vi "ClearListBox.vi"(8 "error in (no error)":errorcluster, 11 "GUI_Handler_Seq in":refnum<class "GUI_Handler_Seq.lvclass">) -> (0 "error out":errorcluster, 3 "GUI_Handler_Seq out":refnum<class "GUI_Handler_Seq.lvclass">)   [LabVIEW 2019, in "GUI_Handler_Seq.lvclass"]
uses:
  GUI_Handler_Seq.lvclass
  <vilib>/Utility/miscctls.llb/LVRowAndColumnTypeDef.ctl
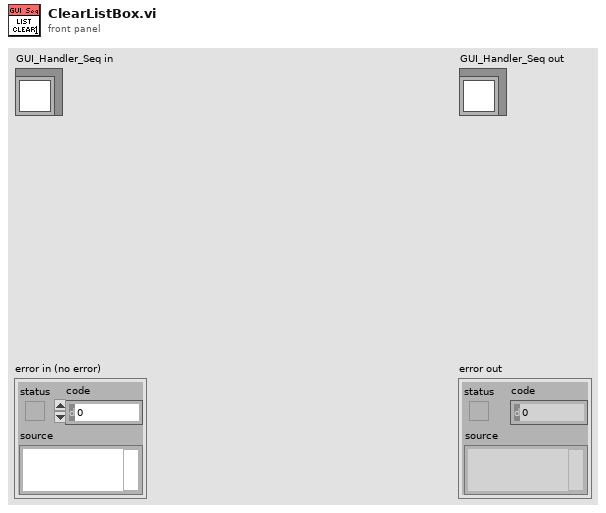
[diagram p1: front panel]
types:
  T1 = typedef "LVRowAndColumnTypeDef.ctl" = cluster{"Row":i32, "Column":i32}
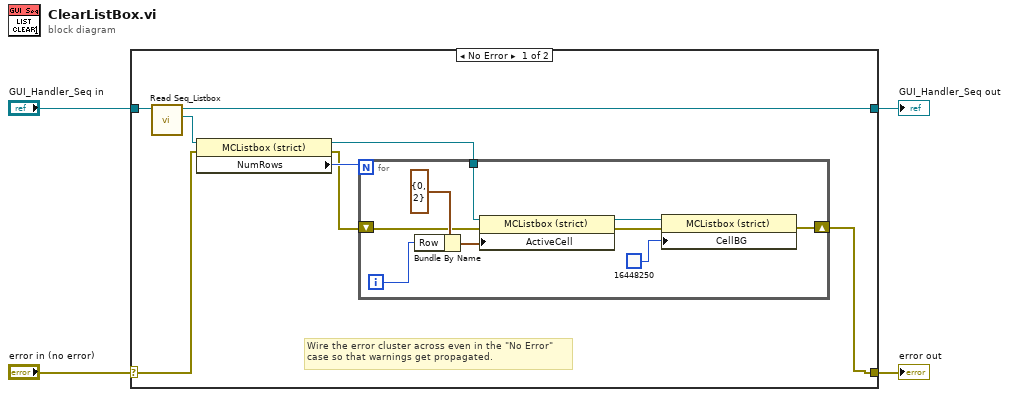
[diagram p0: block diagram]
diagram:
  n1 = case shown="No Error" "error in (no error)" {
    selector: "error in (no error)" -> [w6 w22]
    tunnel: [w5 w22] -> w1
    tunnel: [w12 w23] -> w2
    tunnel: "GUI_Handler_Seq in" -> [w11 w23]
    frame No Error {
      # "Wire the error cluster across even in the \"No Error\"\ncase so that warnings get propagated."
      n2 = call-dynamic "Read Seq_Listbox.vi"("GUI_Handler_Seq in"=w11) -> ("Seq_Listbox"=w10:refnum<vi>, "GUI_Handler_Seq out"=w12:refnum<class "GUI_Handler_Seq.lvclass">)  [unwired: 8 in, 1 out]
      n3 = property class="MCListbox (strict)"(reference=w10, error in=w6) -> (reference out=w8:refnum<vi>, error out=w7:errorcluster, "NumRows"=w9:u32)
      n4 = for {
        N: w9 -> [_]
        tunnel: w8 -> [w18]
        shift-right: [w14] -> w5
        shift-left: w7 -> [w16]
        i -> [w20]
        n5 = Bundle By Name(cluster=T1 {"Row"=0, "Column"=2} ("Active Cell:Active Cell"), "Row"=w20) -> (w19:T1)
        n6 = property class="MCListbox (strict)"(reference=w18, error in=w16, "ActiveCell"=w19) -> (reference out=w17:refnum<vi>, error out=w15:errorcluster)
        n7 = property on="Property Node" class="MCListbox (strict)"(reference=w17, error in=w15, "CellBG"=u32 16448250) -> (error out=w14:errorcluster)  [unwired: 1 out]
      }
    }
    frame Error {
    }
  }
  "error out" <- w1
  "GUI_Handler_Seq out" <- w2
